vi "FSK_Modulation.vi"(0 "PathIn":path, 5 "data":dbl[](array[numeric]), 7 "FreqCarrier1":dbl format="%#_13g", 9 "FreqCarrier2":dbl format="%#_13g", 11 "error in (no error)":errorcluster caption="错误输入（无错误）") -> (4 "PathOut":path, 6 "SendSig":cdb[](array[numeric]) format="%#_13g", 15 "error out":errorcluster caption="错误输出")   [LabVIEW 2015]
panel:
  out "SendSig1 2":dbl[](array[numeric]) format="%#_13g"
  out "SendSig1":dbl[](array[numeric]) format="%#_13g"
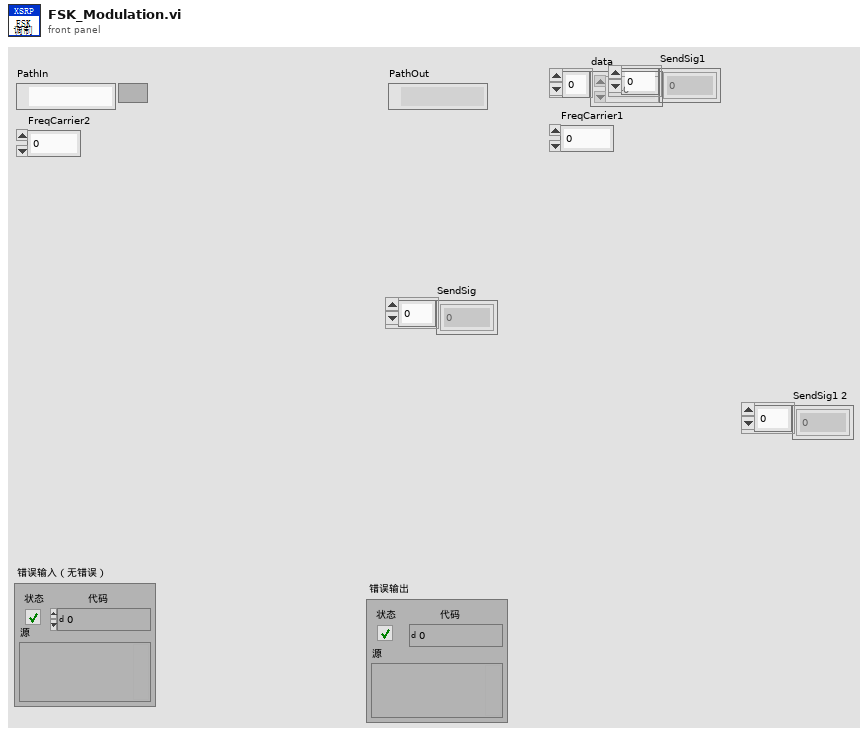
[diagram p1: front panel]
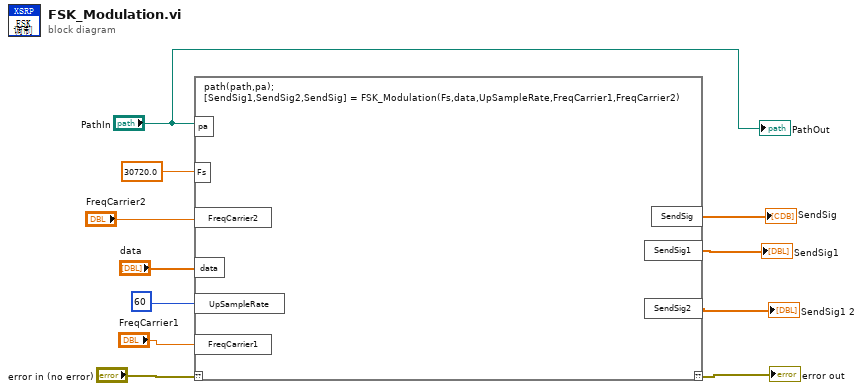
[diagram p0: block diagram]
diagram:
  n1 = script code="path(path,pa);\n[SendSig1,SendSig2,SendSig] = FSK_Modulation(Fs,data,UpSampleRate,FreqCarrier1,FreqCarrier2)"("??"="error in (no error)", "pa"="PathIn", "data"="data", "UpSampleRate"=60, "Fs"=30720.0, "FreqCarrier1"="FreqCarrier1", "FreqCarrier2"="FreqCarrier2") -> ("??"=→"error out":errorcluster, "SendSig"=→"SendSig":cdb[], "SendSig1"=→"SendSig1":dbl[], "SendSig2"=→"SendSig1 2":dbl[])
  "PathOut" <- "PathIn"
